vi "SNMP Get Response.vi"(0 "connection ID":refnum<k16>, 9 "timeout ms (25000)":i32=25000, 11 "error in (no error)":errorcluster) -> (2 "port":u16, 3 "SnmpDataAsStrings":string[][](array[string]), 4 "connection ID out":refnum<k16>, 6 "error-status":i32, 8 "error-string":string, 10 "error-index":i32, 13 "address":i32 format="%.0x", 14 "Req ID":i32, 15 "error out":errorcluster)   [LabVIEW 2017]
doc: "This VI reads the SNMP Get-Response PDU and parses the packet. It will return the data as a multi-dimensional array of strings."
panel:
  out "SNMP Packet":string
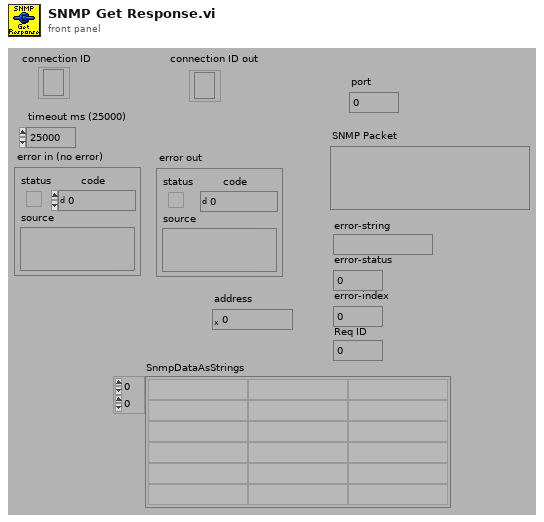
[diagram p1: front panel]
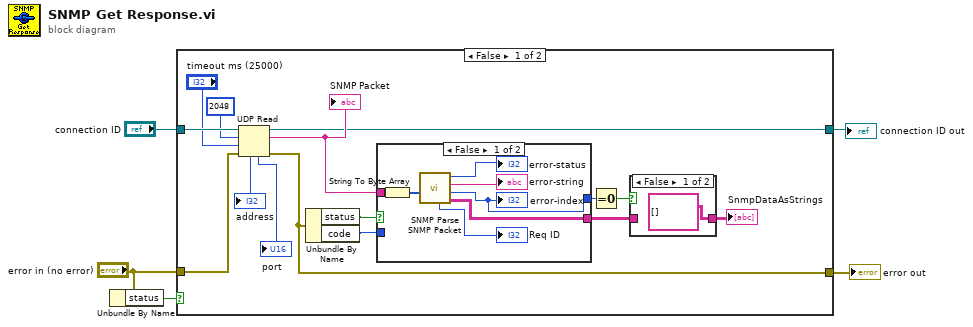
[diagram p0: block diagram]
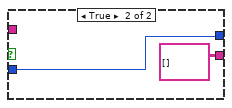
[diagram p2: hidden frame]
diagram:
  n1 = Unbundle By Name("error in (no error)") -> ("status"=w3:bool)
  n2 = case shown="False" w3 {
    tunnel: "connection ID" -> [w17 w32]
    tunnel: "error in (no error)" -> [w14 w33]
    tunnel: [w8 w33] -> w2
    tunnel: [w13 w32] -> w1
    frame False {
      n3 = UDP Read(connection ID=w17, max size (548)=2048, timeout ms (25000)="timeout ms (25000)", 8:w14) -> (data out=w15:string, error out=w8:errorcluster, 3:w13:refnum<k16>, 4:→"port":u16, 6:→"address":u32)
      "SNMP Packet" <- w15
      n4 = Unbundle By Name(w8) -> ("status"=w7:bool, "code"=w6:i32)
      n5 = case shown="False" w7 {
        tunnel: [w27 string[][] [] ("SnmpData")] -> w20
        tunnel: w15 -> [w24 _]
        tunnel: [w21 w28] -> w11
        tunnel: w6 -> [_ w28]
        frame False {
          n6 = String To Byte Array(string=w24) -> (unsigned byte array=w26:u8[])
          n7 = call "SNMP Parse SNMP Packet.vi"("SNMP Packet"=w26) -> ("SnmpData"=w27:string[][], "Error Index"=w21:i32, "Error Status String"=→"error-string":string, "Error Status"=→"error-status":i32, "Req ID"=→"Req ID":i32)  [unwired: 6 out]
          "error-index" <- w21
        }
        frame True {
        }
      }
      n8 = Equal To 0?(x=w11) -> (x = 0?=w12:bool)
      n9 = case shown="False" w12 {
        tunnel: w20 -> [_ w31]
        tunnel: [string[][] [] ("SnmpDataAsStrings") w31] -> w10
        frame False {
        }
        frame True {
        }
      }
      "SnmpDataAsStrings" <- w10
    }
    frame True {
    }
  }
  "error out" <- w2
  "connection ID out" <- w1
